vi "Receive Message.vi"(6 "priority":i32, 10 "Proxy in in":refnum<class "Proxy.lvclass">, 11 "Message in":refnum<class "Message.lvclass">) -> (0 "error out":errorcluster, 2 "Actor out":refnum<class "Actor.lvclass">)   [LabVIEW 2014, in "Proxy.lvlib" / "Proxy.lvclass"]
doc: "This VI should be overriden ONLY if you are creating a proxy actor for remote transmission. If you are, override this VI to transmit the received message to a new destination, maintaining the given priority."
uses:
  Proxy.lvclass
  <vilib>/ActorFramework/Message/Message.lvclass
  <vilib>/ActorFramework/Actor/Actor.lvclass
  Proxy Msg Base/Proxy Msg Base.lvclass
  Proxy.lvclass/Proxy.ctl
  <vilib>/ActorFramework/Message Enqueuer/Message Enqueuer.lvclass/Message Enqueuer.ctl
  <vilib>/ActorFramework/Message Priority Queue/Priority Enqueue.vi
  <vilib>/ActorFramework/Message Enqueuer/Message Enqueuer.lvclass
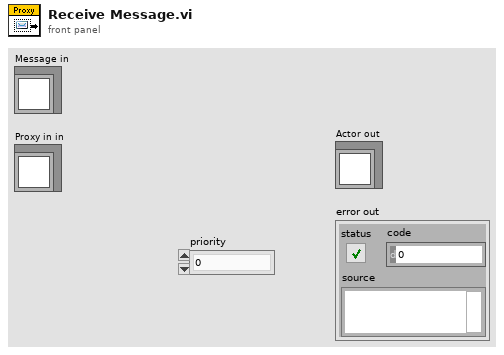
[diagram p1: front panel]
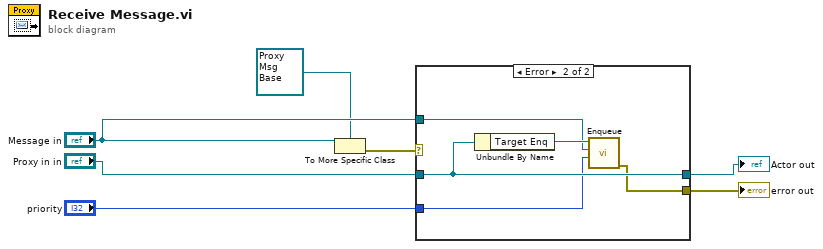
[diagram p0: block diagram]
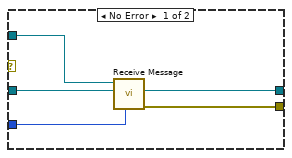
[diagram p2: hidden frame]
diagram:
  n1 = To More Specific Class(target class=refnum<class "Proxy Msg Base.lvclass"> refnum ("Proxy.lvlib:Proxy Msg Base.lvclass"), reference="Message in") -> (error out=w1:errorcluster)  [unwired: 1 in, 1 out]
  n2 = case shown="Error" w1 {
    tunnel: [w12 w13] -> w7
    tunnel: [w11 w17] -> w6
    tunnel: "Proxy in in" -> [w10 w17]
    tunnel: "Message in" -> [w9 w15]
    tunnel: "priority" -> [w8 w14]
    frame No Error {
      n3 = call-parent "Receive Message.vi"("priority"=w8, "Actor in in"=w10, "Message in"=w9) -> ("error out"=w12:errorcluster, "Actor out"=w11:refnum<class "Actor.lvclass">)  [unwired: 7 in]
    }
    frame Error {
      n4 = Unbundle By Name(w17) -> ("Target Enq"=w16:refnum<class "Message Enqueuer.lvclass">)
      n5 = call <vilib>:"Enqueue.vi"("Message Priority (Normal)"=w14, "Message"=w15, "Message Enqueuer in"=w16) -> ("error out"=w13:errorcluster)  [unwired: 7 in, 1 out]
    }
  }
  "error out" <- w7
  "Actor out" <- w6
